vi "DAQmx.Dark.Current.main.vi"() -> ()   [LabVIEW 2020]
uses:
  <vilib>/DAQmx/create/channels.llb/DAQmx Create Channel (DO-Digital Output).vi
panel:
  out "data string 2":string
  out "data string":string
  in  "Clear Pin":tag="Dev1/port0/line0:7"
  in  "Sync Pin":tag="Dev1/port0/line0:7"
  in  "Data Pin":tag="Dev1/port0/line0:7"
  in  "Write Pin":tag="Dev1/port0/line0:7"
  in  "Data to Send":u32[](array[numeric])=[1, 2, 4, 8, 16, 32, 64, 128]
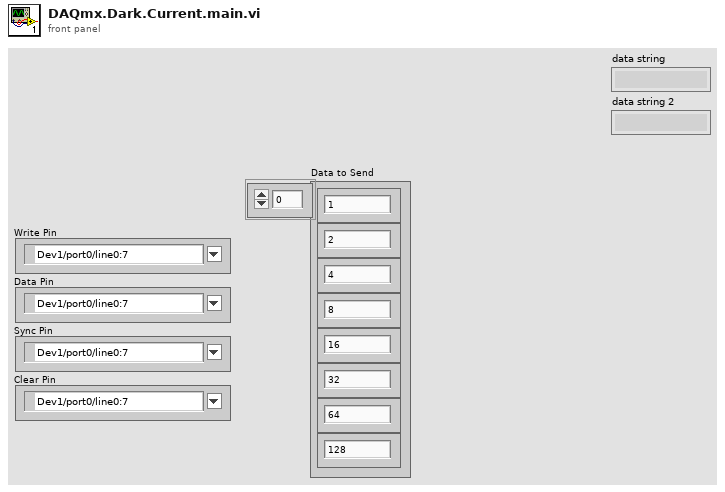
[diagram p1: front panel]
types:
  T1 = cluster{bool, bool, bool, bool, bool, bool, bool, bool}
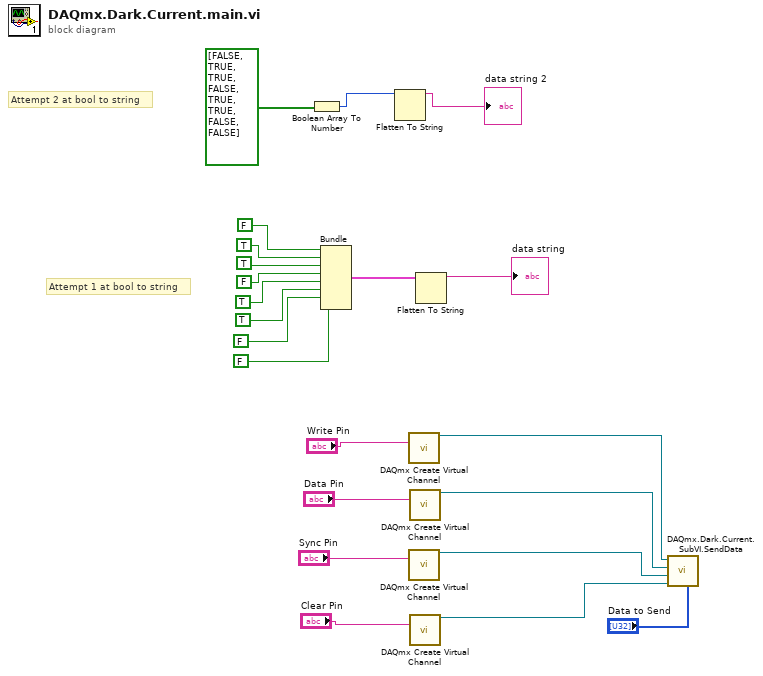
[diagram p0: block diagram]
diagram:
  # "Attempt 2 at bool to string"
  # "Attempt 1 at bool to string"
  n1 = Boolean Array To Number(Boolean array=bool[] [FALSE, TRUE, TRUE, FALSE, TRUE, TRUE, FALSE, FALSE]) -> (number=w1:u32)
  n2 = Bundle(FALSE, TRUE, TRUE, FALSE, TRUE, TRUE, FALSE, FALSE) -> (w12:T1)  [unwired: 1 in]
  n3 = Flatten To String(anything=w1) -> (data string=→"data string 2":string)  [unwired: 3 in, 2 out]
  n4 = call-poly <vilib>:"DAQmx Create Virtual Channel.vi"("lines"="Write Pin") -> ("task out"=w17:refnum<k21>)  [unwired: 13 in, 1 out]
  n5 = call-poly <vilib>:"DAQmx Create Virtual Channel.vi"("lines"="Sync Pin") -> ("task out"=w15:refnum<k21>)  [unwired: 13 in, 1 out]
  n6 = call-poly <vilib>:"DAQmx Create Virtual Channel.vi"("lines"="Data Pin") -> ("task out"=w16:refnum<k21>)  [unwired: 13 in, 1 out]
  n7 = call-poly <vilib>:"DAQmx Create Virtual Channel.vi"("lines"="Clear Pin") -> ("task out"=w14:refnum<k21>)  [unwired: 13 in, 1 out]
  n8 = Flatten To String(anything=w12) -> (data string=→"data string":string)  [unwired: 3 in, 2 out]
  n9 = call "DAQmx.Dark.Current.SubVI.SendData.vi"("Write Pin Task In"=w17, "Data Pin Task In"=w16, "Sync Pin Task In"=w15, "Clear Pin Task In"=w14, "Data to Send in"="Data to Send") -> ()  [unwired: 1 in, 4 out]
